vi "Periodic Tasks.vi"(8 "error in":errorcluster) -> ()   [LabVIEW 2013]
doc: "This VI runs in parallel to other tasks. It can contain as many user-defined periodic loops as you need. These can carry out PID or other sorts of timed response."
uses:
  RefnameEnum.ctl
  <vilib>/Rock Robotics/SystemInterfaces/Utilities/FPGA_UtilitiesLED Source.ctl
  <vilib>/Rock Robotics/SystemInterfaces/Utilities/FPGA_UtilitiesLED State.ctl
  <vilib>/Rock Robotics/WPI/Compressor/WPI_CompressorGetSetRefNum.vi
  Robot Global Data.vi
panel:
  out "Compressor Loop Running":bool
  out "Compressor Running":bool
  out "Compressor Enabled":bool
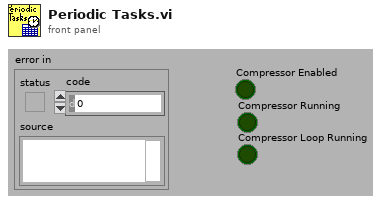
[diagram p1: front panel]
types:
  T1 = typedef "RefnameEnum.ctl" = enum16{"FireLauncher", "Climber", "Shield", "TankDrive", "DriveEncoderL", "DriveEncoderR", "LauncherMotorRPM", "LauncherEncoderAnalog", "LauncherEncoderRPM", "ShooterLS", "DriveAlignLSLeft", "DriveAlignLSRight", "ClimbingLS", "LauncherEncoderAngle", "LauncherMotorAngle", "Gamepad1", "Gamepad2", "Compressor", "ClimbWeightSol3", "ClimbWeightSol4"}
  T2 = typedef "FPGA_UtilitiesLED State.ctl" = enum16{"Off", "On", "Toggle"}
  T3 = typedef "FPGA_UtilitiesLED Source.ctl" = enum16{"User LED", "FPGA LED"}
  T4 = typedef "WPI_CompressorDevRef.ctl" = cluster{"DevStatus":errorcluster, "DigitalInputDevRef":T5, "RelayDevRef":T8}
  T5 = typedef "WPI_DigitalInputDevRef.ctl" = cluster{"DevStatus":errorcluster, "DIO Channel":T6, "Digital Module":T7}
  T6 = typedef "FPGA_DIOChannel.ctl" = enum8{"DIO 1", "DIO 2", "DIO 3", "DIO 4", "DIO 5", "DIO 6", "DIO 7", "DIO 8", "DIO 9", "DIO 10", "DIO 11", "DIO 12", "DIO 13", "DIO 14", "Invalid"}
  T7 = typedef "FPGA_TypedefDigitalModule.ctl" = enum16{"Digital Module 1", "Digital Module 2"}
  T8 = typedef "WPI_RelayDevRef.ctl" = cluster{"DevStatus":errorcluster, "Relay Channel":T9, "Digital Module":T7, "Relay Direction":T10}
  T9 = typedef "FPGA_DIORelayChannel.ctl" = enum8{"Relay 1", "Relay 2", "Relay 3", "Relay 4", "Relay 5", "Relay 6", "Relay 7", "Relay 8", "Invalid"}
  T10 = typedef "WPI_RelayDirection.ctl" = enum16{"Both directions", "Forward only", "Reverse only"}
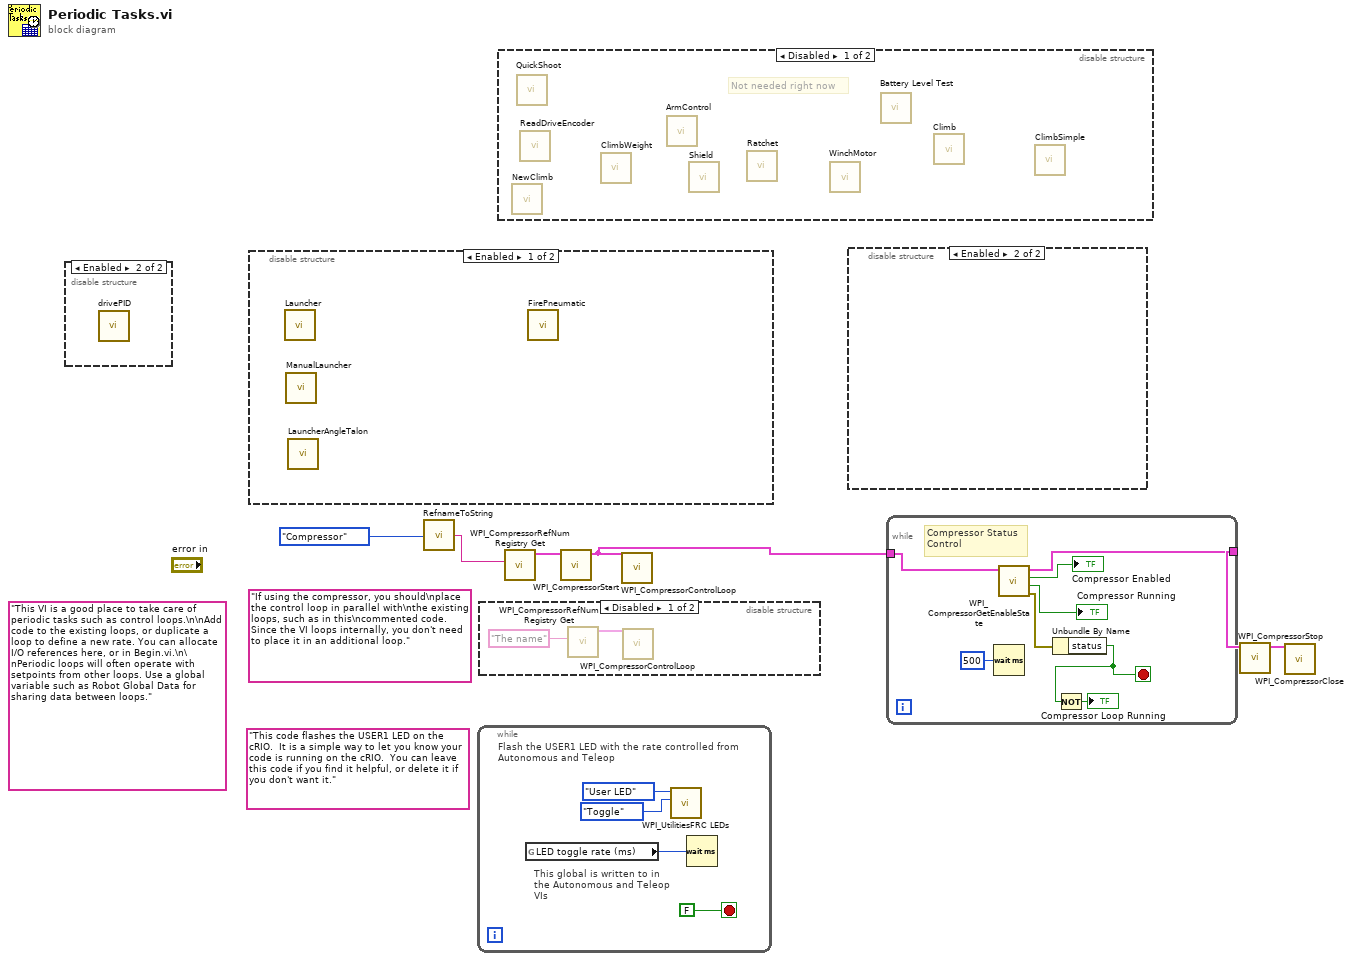
[diagram p0: block diagram]
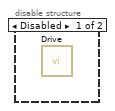
[diagram p2: hidden frame]
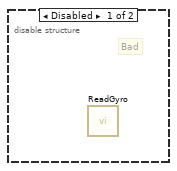
[diagram p4: hidden frame]
diagram:
  (unwired) "If using the compressor, you should\nplace the control loop in parallel with\nthe existing loops, such as in this\ncommented code. Since the VI loops internally, you don't need to place it in an additional loop."
  (unwired) "This code flashes the USER1 LED on the cRIO.  It is a simple way to let you know your code is running on the cRIO.  You can leave this code if you find it helpful, or delete it if you don't want it."
  (unwired) "This VI is a good place to take care of periodic tasks such as control loops.\n\nAdd code to the existing loops, or duplicate a loop to define a new rate. You can allocate I/O references here, or in Begin.vi.\n\nPeriodic loops will often operate with setpoints from other loops. Use a global variable such as Robot Global Data for sharing data between loops."
  n1 = disable-structure shown="Enabled" {
    frame Disabled {
      n2 = call "Drive.vi"() -> ()  [unwired: 12 in]
    }
    frame Enabled {
      n3 = call "drivePID.vi"() -> ()  [unwired: 12 in]
    }
  }
  n4 = disable-structure shown="Enabled" {
    frame Enabled {
      n5 = call "Launcher.vi"() -> ()  [unwired: 12 in]
      n6 = call "ManualLauncher.vi"() -> ()  [unwired: 12 in]
      n7 = call "LauncherAngleTalon.vi"() -> ()  [unwired: 12 in]
      n8 = call "FirePneumatic.vi"() -> ()  [unwired: 12 in]
    }
    frame Disabled {
    }
  }
  n9 = call "RefnameToString.vi"("Enum"=RefnameEnum."Compressor") -> ("Refname"=w1:string)
  n10 = while {
    stop <- FALSE stop-if-true
    # "This global is written to in the Autonomous and Teleop VIs"
    # "Flash the USER1 LED with the rate controlled from Autonomous and Teleop"
    n11 = global read "Robot Global Data.vi" "LED toggle rate (ms)"() -> (w7:u32)
    n12 = call <vilib>:"WPI_UtilitiesFRC LEDs.vi"("State"=FPGA_UtilitiesLED_State."Toggle", "LED Type"=FPGA_UtilitiesLED_Source."User LED") -> ()  [unwired: 1 in, 9 out]
    n13 = Wait (ms)(milliseconds to wait=w7) -> ()  [unwired: 1 out]
  }
  n14 = disable-structure shown="Disabled" {
    frame Disabled {
      n15 = call <vilib>:"WPI_CompressorRefNum Registry Get.vi"("refnum name"="The name") -> ("CompressorDevRef"=w12:T4)  [unwired: 9 in, 1 out]
      n16 = call <vilib>:"WPI_CompressorControlLoop.vi"("CompressorDevRef"=w12) -> ()  [unwired: 11 in]
    }
    frame Enabled {
    }
  }
  n17 = disable-structure shown="Disabled" {
    frame Disabled {
      # "Not needed right now"
      n18 = call "NewClimb.vi"() -> ()  [unwired: 12 in]
      n19 = call "QuickShoot.vi"() -> ()  [unwired: 12 in]
      n20 = call "ReadDriveEncoder.vi"() -> ()  [unwired: 12 in]
      n21 = call "ClimbWeight.vi"() -> ()  [unwired: 12 in]
      n22 = call "ArmControl.vi"() -> ()  [unwired: 12 in]
      n23 = call "Shield.vi"() -> ()  [unwired: 12 in]
      n24 = call "Ratchet.vi"() -> ()  [unwired: 12 in]
      n25 = call "WinchMotor.vi"() -> ()  [unwired: 12 in]
      n26 = call "Battery Level Test.vi"() -> ()  [unwired: 12 in]
      n27 = call "Climb.vi"() -> ()  [unwired: 12 in]
      n28 = call "ClimbSimple.vi"() -> ()  [unwired: 12 in]
    }
    frame Enabled {
    }
  }
  n29 = call <vilib>:"WPI_CompressorRefNum Registry Get.vi"("refnum name"=w1) -> ("CompressorDevRef"=w6:T4)  [unwired: 9 in, 1 out]
  n30 = call <vilib>:"WPI_CompressorStart.vi"("CompressorDevRef"=w6) -> ("CompressorDevRef"=w5:T4)  [unwired: 9 in, 1 out]
  n31 = call <vilib>:"WPI_CompressorControlLoop.vi"("CompressorDevRef"=w5) -> ()  [unwired: 11 in]
  n32 = disable-structure shown="Enabled" {
    frame Disabled {
      # "Bad"
      n33 = call "ReadGyro.vi"() -> ()  [unwired: 12 in]
    }
    frame Enabled {
    }
  }
  n34 = while {
    tunnel: w5 -> [w20]
    tunnel: [w15] -> w4
    stop <- w13 stop-if-true
    # "Compressor Status\nControl"
    n35 = Wait (ms)(milliseconds to wait=u32 500) -> ()  [unwired: 1 out]
    n36 = call <vilib>:"WPI_CompressorGetEnableState.vi"("CompressorDevRef"=w20) -> ("error out"=w16:errorcluster, "Compressor Running"=→"Compressor Running":bool, "Enabled"=→"Compressor Enabled":bool, "CompressorDevRef"=w15:T4)  [unwired: 1 in, 6 out]
    n37 = Unbundle By Name(w16) -> ("status"=w13:bool)
    n38 = Not(x=w13) -> (.not. x?=→"Compressor Loop Running":bool)
  }
  n39 = call <vilib>:"WPI_CompressorStop.vi"("CompressorDevRef"=w4) -> ("CompressorDevRef"=w3:T4)  [unwired: 1 in, 9 out]
  n40 = call <vilib>:"WPI_CompressorClose.vi"("CompressorDevRef"=w3) -> ()  [unwired: 1 in, 10 out]
